vi "Global Constants.vi"() -> ()   [LabVIEW 2018]
panel:
  in  "manipLength":dbl
  in  "foreArmLength":dbl
  in  "bicepLength":dbl
  in  "Yaw acceptable turn range":dbl=5.0
  in  "Drive Loop Iteration Time":dbl=5.0
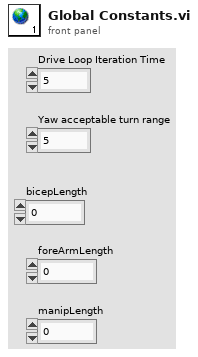
[diagram p1: front panel]
diagram:
